vi "Continuous Camera Test.vi"() -> ()   [LabVIEW 2017]
uses:
  <vilib>/Platform/TimedLoop/XDataNode/timing_clust.ctl
  <vilib>/Platform/TimedLoop/XDataNode/nitl_modes.ctl
  <vilib>/Platform/TimedLoop/XDataNode/wakeup.ctl
  <vilib>/Platform/TimedLoop/XDataNode/XDataNode.xnode
  IMAQCV/IMAQCV.lvlib
  <vilib>/Platform/TimedLoop/XDataNode/XDNodeRunTimeDep.lvlib
  IMAQCV/PIIO.lvlib
panel:
  out "Loop Rate (Hz)":u32
  in  "stop":bool
  in  "Image Size":T1(ring)=enum."640 (H)   x  480 (V) "
  in  "type":enum16{"GRAY", "COLOR"}(ring)=enum."COLOR"
  out "picture":picture
  out "error out":errorcluster
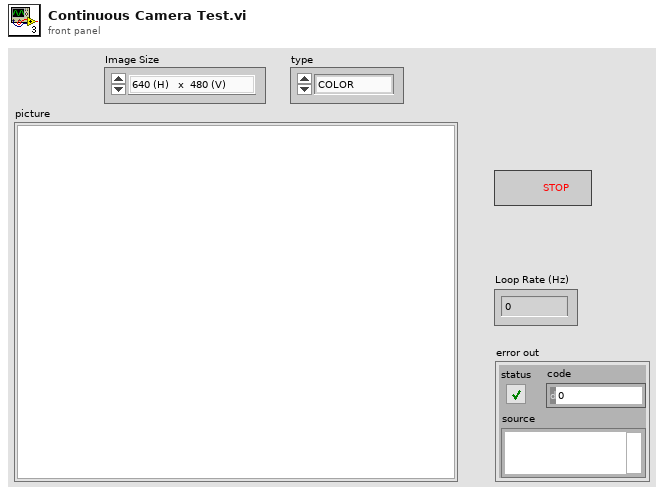
[diagram p1: front panel]
types:
  T1 = enum16{"320 (H)   x  240 (V)", "352(H)    x  288 (V)", "640 (H)   x  480 (V) ", "800 (H)   x  600 (V)", "1024 (H) x  768 (V)", "1280 (H) x  720 (V)", "1280 (H) x  960 (V)", "1280 (H) x 1024 (V)", "1920 (H) x 1080 (V)"}
  T2 = typedef "IMAQCV.lvlib/IMAQCV Image.ctl" = refnum<vi>
  T3 = typedef "XDNodeRunTimeDep.lvlib/timing_clust.ctl" = cluster{"Expected End [f-1]":u64, "Actual End [f-1]":u64, "Finished Late? [f-1]":bool, "Expected End [i-1]":u64, "Actual End [i-1]":u64, "Finished Late? [i-1]":bool, "Expected Start [i]":u64, "Actual Start [i]":u64, "Expected Start [f]":u64, "Actual Start [f]":u64, "Source Name":string, "Structure Name":string, "Period":i64, "Deadline":i64, "Offset":i64, "Start":i64, "Priority":i32, "Timeout":i32, "Mode":T4, "Wakeup Reason":T5, "Error":errorcluster, "Source Type":string, "Secondary Source Type":string, "Global End Time":u64, "Global Start Time":u64, "Frame Duration":u64, "Iteration Duration":u64, "Assigned CPU":i32, "I/O Scan Engine Mode":u32}
  T4 = typedef "XDNodeRunTimeDep.lvlib/nitl_modes.ctl" = enum32{"No Change", "Process missed periods, maintain original phase", "Discard missed periods, maintain original phase", "Process missed periods, ignore original phase", "Discard missed periods, ignore original phase"}
  T5 = typedef "XDNodeRunTimeDep.lvlib/wakeup.ctl" = enum32{"Normal", "Aborted", "Asynchronous wakeup", "Timing source error", "Timed loop error", "Timeout"}
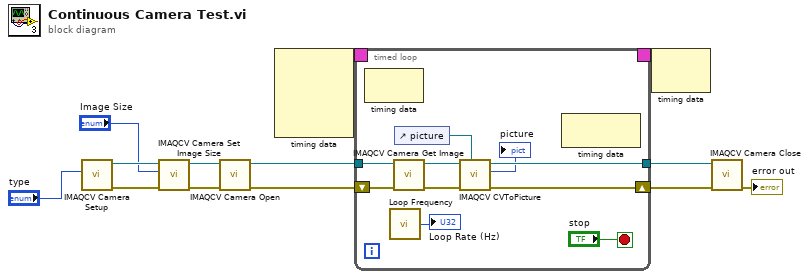
[diagram p0: block diagram]
diagram:
  n1 = call "IMAQCV Camera Setup.vi"("type"="type") -> ("error out"=w13:errorcluster, "image out"=w9:T2)  [unwired: 9 in]
  n2 = call "IMAQCV Camera Set Image Size.vi"("error in (no error)"=w13, "Image Size"="Image Size", "image in"=w9) -> ("error out"=w4:errorcluster, "image out"=w3:T2)  [unwired: 7 in]
  n3 = call "IMAQCV Camera Open.vi"("error in (no error)"=w4, "image in"=w3) -> ("error out"=w12:errorcluster, "image out"=w8:T2)  [unwired: 8 in]
  n4 = node-c288() -> (w2:T3)  [unwired: 4 in]
  n5 = timed-loop {
    shift-right: [w21] -> w11
    shift-left: w12 -> [w23]
    tunnel: w8 -> [w20]
    tunnel: [w18] -> w7
    timing: w2 -> [_]
    timing-out: [_] -> w1
    stop <- "stop" stop-if-true
    n6 = node-c288() -> ()  [unwired: 1 in, 1 out]
    n7 = call "Loop Frequency.vi"() -> ("Loop Rate (Hz)"=→"Loop Rate (Hz)":u32)  [unwired: 1 out]
    n8 = call "IMAQCV Camera Get Image.vi"("error in (no error)"=w23, "image in"=w20) -> ("error out"=w22:errorcluster, "image out"=w19:T2)  [unwired: 8 in]
    n9 = control-ref of="picture"() -> (w16:refnum<vi>)
    n10 = call "IMAQCV CVToPicture.vi"("picture ref"=w16, "error in (no error)"=w22, "image"=w19) -> ("error out"=w21:errorcluster, "picture"=→"picture":picture, "image out"=w18:T2)  [unwired: 6 in]
    n11 = node-c288() -> ()  [unwired: 1 in, 1 out]
  }
  n12 = node-c288(w1) -> ()  [unwired: 1 out]
  n13 = call "IMAQCV Camera Close.vi"("error in (no error)"=w11, "Image"=w7) -> ("error out"=→"error out":errorcluster)  [unwired: 9 in]
